vi "YSCS_ADD8.vi"(1 "结束位置":u32, 2 "校验起始位":u32, 3 "输入字符串":string) -> (0 "输出字符串":string)   [LabVIEW 2015]
doc: "校验和，将数据累加起来，取低8位"
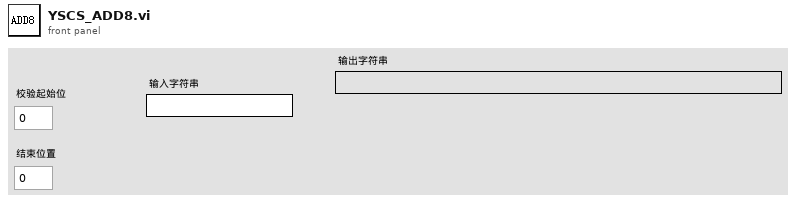
[diagram p1: front panel]
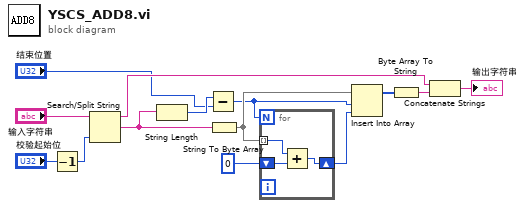
[diagram p0: block diagram]
diagram:
  n1 = Decrement(x="校验起始位") -> (x-1=w11:u32)
  n2 = Search/Split String(string="输入字符串", offset (0)=w11) -> (substring before match=w10:string, match + rest of string=w4:string)  [unwired: 1 in, 1 out]
  n3 = String Length(string=w4) -> (length=w3:i32)
  n4 = Subtract(x=w3, y="结束位置") -> (x-y=w1:u32)
  n5 = String To Byte Array(string=w4) -> (unsigned byte array=w7:u8[])
  n6 = for {
    N: w1 -> [_]
    tunnel: w7 -> [w15] mode=indexing
    shift-right: [w17] -> w5
    shift-left: u8 0 -> [w16]
    n7 = Add(x=w15, y=w16) -> (x+y=w17:u8)
  }
  n8 = Insert Into Array(array=w7, index=w1, new element=w5) -> (w6:u8[])
  n9 = Byte Array To String(unsigned byte array=w6) -> (string=w9:string)
  n10 = Concatenate Strings(w10, w9) -> (→"输出字符串":string)
